vi "Destroy to SSH.vi"(8 "Error In":errorcluster, 11 "SFTP Attributes":refnum<class "File Info.lvclass">) -> (0 "Error Out":errorcluster, 3 "SSH":refnum<class "SSH.lvclass">)   [LabVIEW 2018, in "Toolkit.lvlib" / "File Info.lvclass"]
uses:
  File Info.lvclass
  Toolkit.lvlib
  SSH/SSH.lvclass
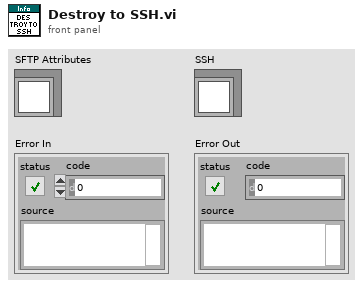
[diagram p1: front panel]
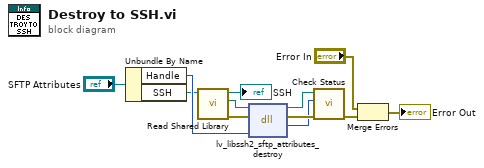
[diagram p0: block diagram]
diagram:
  n1 = Unbundle By Name("SFTP Attributes") -> ("Handle"=w10:u64, "SSH"=w4:refnum<class "SSH.lvclass">)
  n2 = call "Read Shared Library.vi"("SSH In"=w4) -> ("Error Out"=w3:errorcluster, "lv-libssh2 Shared Library"=w2:path, "SSH Out"=→"SSH":refnum<class "SSH.lvclass">)  [unwired: 8 in]
  n3 = dll-call lib="lv-libssh2.*" fn="lv_libssh2_sftp_attributes_destroy"(path in=w2, error in=w3, "handle"=w10) -> (path out=w8:path, error out=w9:errorcluster, "status"=w7:i32)  [unwired: 2 in]
  n4 = call "Check Status.vi"("Error In"=w9, "Status"=w7, "lv-libssh2 Shared Library In"=w8) -> ("Error Out"=w6:errorcluster)  [unwired: 7 in, 1 out]
  n5 = Merge Errors("Error In", w6) -> (→"Error Out":errorcluster)
